vi "UnpackFieldsFromBuffer.vi"(8 "error in (no error)":errorcluster, 11 "Buffer":u8[](array[numeric])) -> (0 "error out":errorcluster, 3 "Fields Ref Out":T1)   [LabVIEW 2019, in "Template Server.lvlib" / "gprc-lvsupport.lvlib"]
uses:
  gprc-lvsupport.lvlib
  typeDefs/grpcId.ctl
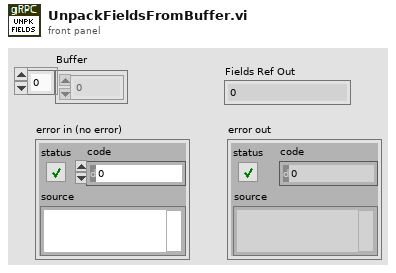
[diagram p1: front panel]
types:
  T1 = typedef "Template Server.lvlib/gprc-lvsupport.lvlib/grpcId.ctl" = u64
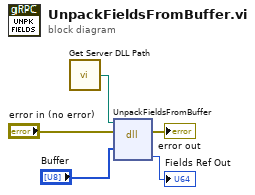
[diagram p0: block diagram]
diagram:
  n1 = call "Get Server DLL Path.vi"() -> ("Server dll path"=w4:path)
  n2 = dll-call lib="?" fn="UnpackFieldsFromBuffer"(path in=w4, error in="error in (no error)", "buffer"="Buffer") -> (error out=→"error out":errorcluster, "elementRef"=→"Fields Ref Out":u64)  [unwired: 4 in, 1 out]
